vi "ServoMoveTimeWrite.vi"(8 "Time":u16=1000 max=30000 step=1, 9 "Angel":dbl min=0.0 max=240.0 step=0.24, 10 "ID":u8=1) -> (2 "Command":string)   [LabVIEW 2013]
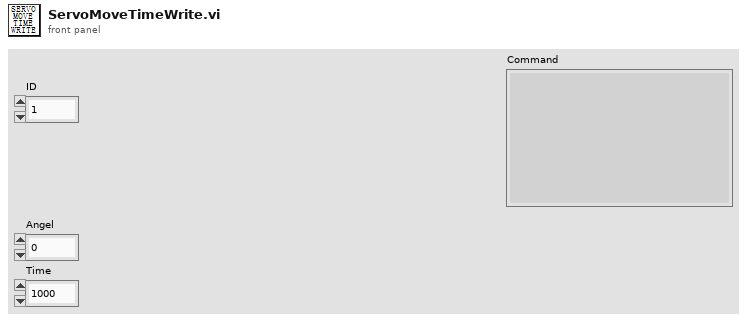
[diagram p1: front panel]
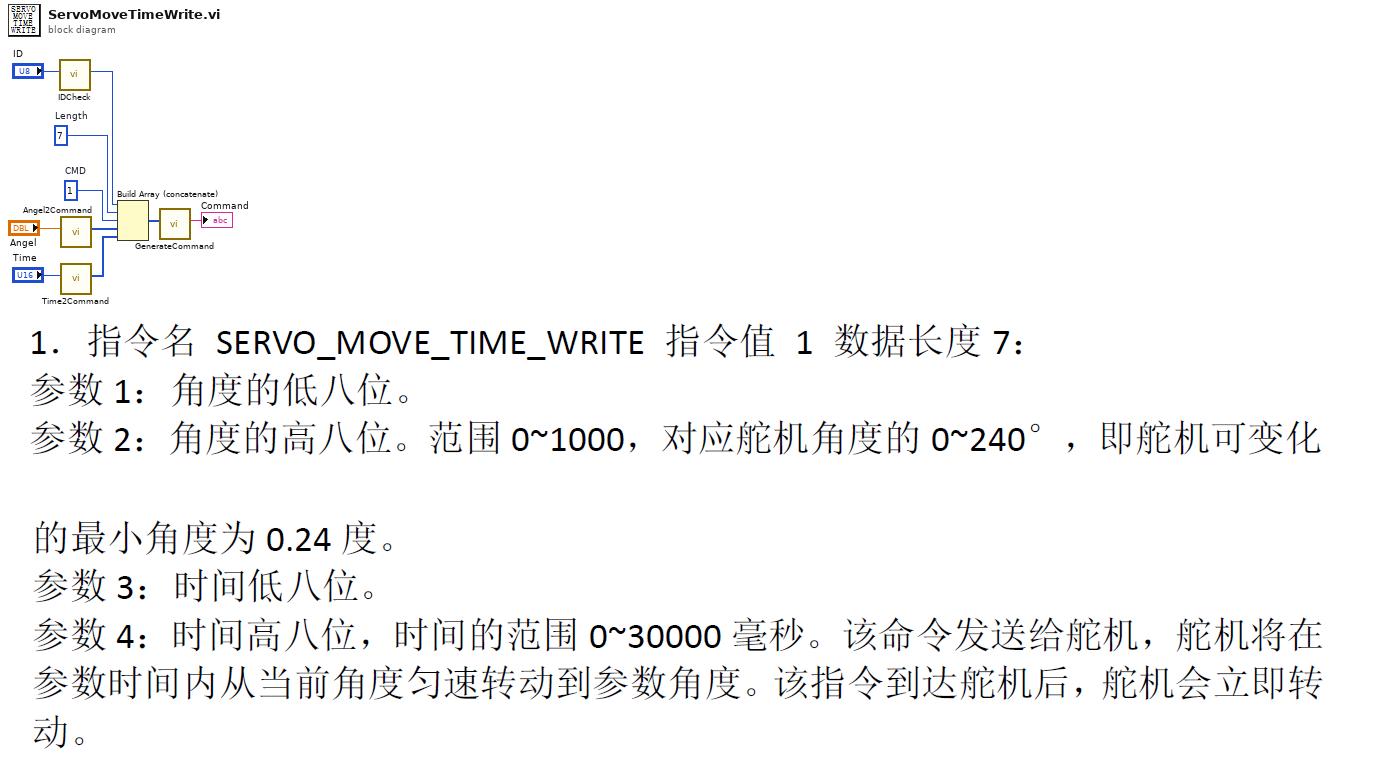
[diagram p0: block diagram]
diagram:
  w5 = u8 1  # CMD
  w6 = u8 7  # Length
  n1 = call "IDCheck.vi"("IDIn"="ID") -> ("IDOut"=w7:u8)  [unwired: 10 in]
  n2 = call "Angel2Command.vi"("AngelIn"="Angel") -> ("CommandOut"=w4:u8[])  [unwired: 10 in]
  n3 = call "Time2Command.vi"("TimeIn"="Time") -> ("CommandOut"=w3:u8[])  [unwired: 10 in]
  n4 = Build Array (concatenate)(w7, w6, w5, w4, w3) -> (w2:u8[])
  n5 = call "GenerateCommand.vi"("DataIn"=w2) -> ("Command"=→"Command":string)  [unwired: 10 in]
